vi "Test.vi"() -> ()   [LabVIEW 2010]
uses:
  <vilib>/Utility/NIReport.llb/NI_report.lvclass
  <vilib>/Utility/NIReport.llb/Append Report Text (str wrap).vi
  <vilib>/measure/NI_MABase.lvlib
panel:
  out "File path":path
  out "Waveform Graph":waveform(dbl)(graph)
  in  "Save Filename":string="zzxx3.pdf"
  in  "Save Directory":path=path "C:/tmp"
  in  "printer name (default) or file path (dialog)":string="PDFCreator"
  in  "report type":T1(ring)
  in  "font settings":T2={"charset (-1)"=-1, "weight (-1)"=-1, "name"="", "size"=" "}
  in  "orientation (portrait)":u16(ring) items=["portrait", "landscape"]
  in  "footers":T3
  in  "margins":T4={"margins (1.00)"={"top"=1.0, "left"=1.0, "right"=1.0, "bottom"=1.0}, "measurement system (default)"=0} {"measurement system (default)" items=["Default", "US", "Metric"]; "margins (1.00)"."right" format="%0.2f"; "margins (1.00)"."bottom" format="%0.2f"; "margins (1.00)"."top" format="%0.2f"; "margins (1.00)"."left" format="%0.2f"}
  in  "headers":T3
  out "error out":errorcluster
  in  "error in (no error)":errorcluster
  in  "text to be printed":string="TEST\nTEST\nTEST\nTEST\nTEST\nTEST\n"
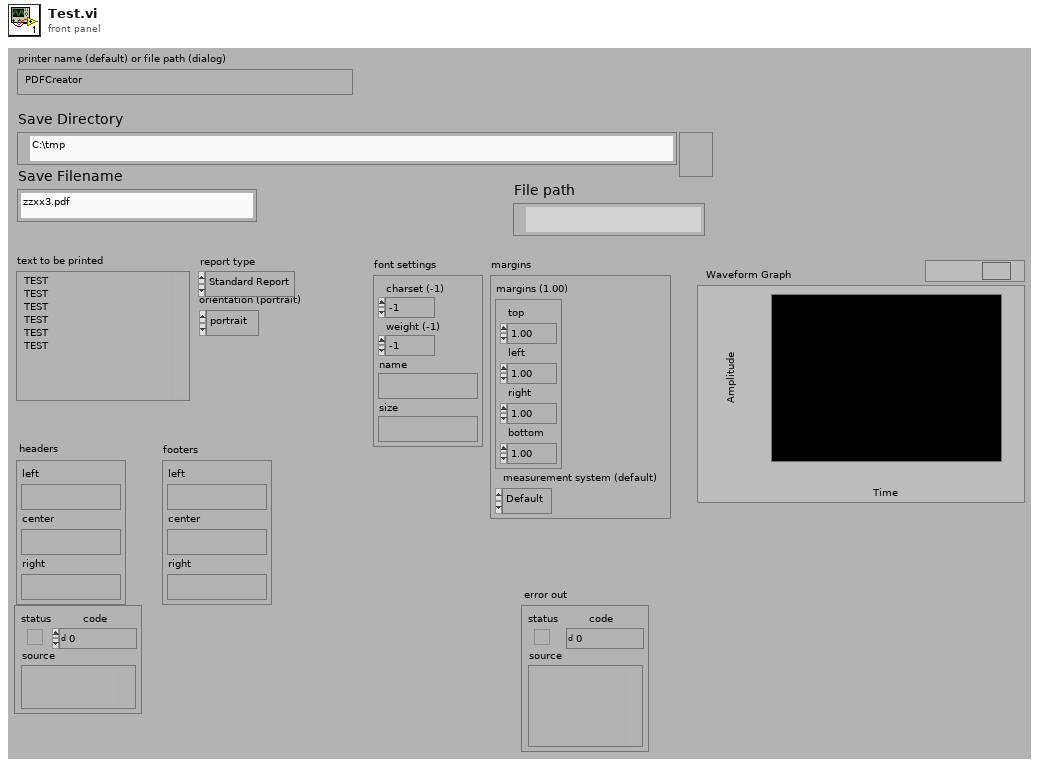
[diagram p1: front panel]
types:
  T1 = enum16{"Standard Report", "HTML", "Word", "Excel"}
  T2 = cluster{"charset (-1)":i16, "weight (-1)":i16, "name":string, "size":string}
  T3 = cluster{"left":string, "center":string, "right":string}
  T4 = cluster{"margins (1.00)":cluster{"top":dbl, "left":dbl, "right":dbl, "bottom":dbl}, "measurement system (default)":u16}
  T5 = cluster{"frequency":dbl, "amplitude":dbl, "phase":dbl}[]
  T6 = cluster{"top":dbl, "left":dbl, "right":dbl, "bottom":dbl}
  T7 = typedef "imagedata.ctl" = cluster{"image type":i32, "image depth":i32, "image":u8[], "mask":u8[], "colors":u32[], "Rectangle":cluster{"left":i16, "top":i16, "right":i16, "bottom":i16}}
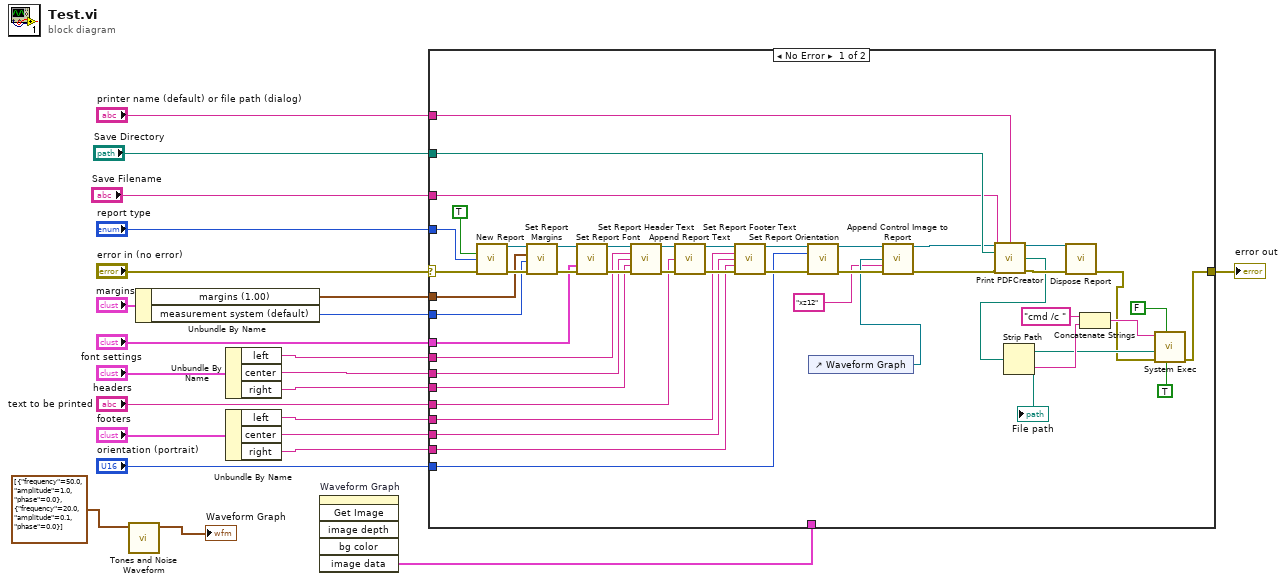
[diagram p0: block diagram]
diagram:
  n1 = call <vilib>:"Tones and Noise Waveform.vi"("tones"=T5 [{"frequency"=50.0, "amplitude"=1.0, "phase"=0.0}, {"frequency"=20.0, "amplitude"=0.1, "phase"=0.0}]) -> ("signal out"=→"Waveform Graph":waveform(dbl))  [unwired: 9 in, 1 out]
  n2 = Unbundle By Name("margins") -> ("margins (1.00)"=w21:T6, "measurement system (default)"=w20:u16)
  n3 = Unbundle By Name("headers") -> ("left"=w18:string, "center"=w17:string, "right"=w16:string)
  n4 = Unbundle By Name("footers") -> ("left"=w14:string, "center"=w13:string, "right"=w12:string)
  n5 = invoke on="Waveform Graph" class="WFGraph (strict)" method="Get Image"() -> ("image data"=w1:T7)  [unwired: 6 in, 5 out]
  n6 = case shown="No Error" "error in (no error)" {
    selector: "error in (no error)" -> [w58 w69]
    tunnel: [w24 w69] -> w23
    tunnel: w21 -> [w66 _]
    tunnel: w20 -> [w63 _]
    tunnel: w18 -> [w55 _]
    tunnel: w17 -> [w62 _]
    tunnel: w16 -> [w61 _]
    tunnel: w14 -> [w51 _]
    tunnel: w13 -> [w49 _]
    tunnel: w12 -> [w50 _]
    tunnel: "text to be printed" -> [w48 _]
    tunnel: "orientation (portrait)" -> [w44 _]
    tunnel: "font settings" -> [w47 _]
    tunnel: "report type" -> [w43 _]
    tunnel: "printer name (default) or file path (dialog)" -> [w40 _]
    tunnel: "Save Directory" -> [w39 _]
    tunnel: "Save Filename" -> [w38 _]
    tunnel: w1 -> [_ _]
    frame No Error {
      n7 = call <vilib>:"New Report.vi"("display alerts? (F)"=TRUE, "report type"=w43, "error in (no error)"=w58) -> ("report out"=w68:refnum<class "NI_report.lvclass">, "error out"=w67:errorcluster)  [unwired: 3 in, 8 out]
      n8 = call-dynamic "Set Report Margins.vi"("report in"=w68, "margins (1.00)"=w66, "measurement system (default)"=w63, "error in (no error)"=w67) -> ("report out"=w60:refnum<class "NI_report.lvclass">, "error out"=w59:errorcluster)  [unwired: 10 out]
      n9 = call-dynamic "Set Report Font.vi"("report in"=w60, "font settings"=w47, "error in (no error)"=w59) -> ("report out"=w65:refnum<class "NI_report.lvclass">, "error out"=w64:errorcluster)  [unwired: 3 in, 8 out]
      n10 = call-dynamic "Set Report Header Text.vi"("report in"=w65, "left header text"=w55, "center header text"=w62, "right header text"=w61, "error in (no error)"=w64) -> ("report out"=w57:refnum<class "NI_report.lvclass">, "error out"=w52:errorcluster)  [unwired: 2 in, 7 out]
      n11 = call-poly <vilib>:"Append Report Text.vi"("report in"=w57, "text"=w48, "error in (no error)"=w52) -> ("report out"=w56:refnum<class "NI_report.lvclass">, "error out"=w53:errorcluster)  [unwired: 3 in, 8 out]
      n12 = call-dynamic "Set Report Footer Text.vi"("report in"=w56, "left footer text"=w51, "center footer text"=w49, "right footer text"=w50, "error in (no error)"=w53) -> ("report out"=w46:refnum<class "NI_report.lvclass">, "error out"=w45:errorcluster)  [unwired: 1 in, 8 out]
      n13 = call-dynamic "Set Report Orientation.vi"("report in"=w46, "orientation (portrait)"=w44, "error in (no error)"=w45) -> ("report out"=w37:refnum<class "NI_report.lvclass">, "error out"=w36:errorcluster)  [unwired: 11 out]
      n14 = control-ref of="Waveform Graph"() -> (w34:refnum<vi>)
      n15 = call-dynamic "Append Control Image to Report.vi"("report in"=w37, "ctrl reference"=w34, "description"="xz12") -> ("report out"=w35:refnum<class "NI_report.lvclass">)  [unwired: 9 in, 3 out]
      n16 = call "Print PDFCreator.vi"("report in"=w35, "Printer name"=w40, "Save Directory"=w39, "Save Filename"=w38, "error in (no error)"=w36) -> ("report out"=w41:refnum<class "NI_report.lvclass">, "File path"=w26:path, "error out"=w42:errorcluster)  [unwired: 8 out]
      "File path" <- w26
      n17 = Strip Path(path=w26) -> (stripped path=w29:path, name=w30:string)
      n18 = call-dynamic "Dispose Report.vi"("report in"=w41, "error in (no error)"=w42) -> ("error out"=w25:errorcluster)  [unwired: 3 in, 10 out]
      n19 = Concatenate Strings("cmd /c " ("string"), w30) -> (w31:string)
      n20 = call <vilib>:"System Exec.vi"("run minimized? (F)"=TRUE, "wait until completion? (T)"=FALSE, "error in (no error)"=w25, "working directory"=w29, "command line"=w31) -> ("error out"=w24:errorcluster)  [unwired: 3 in, 3 out]
    }
    frame Error {
    }
  }
  "error out" <- w23
